vi "Initialize_Msg_Queue_FGV.vi"(8 "error in (no error)":errorcluster, 11 "queue Out":refnum<queue>) -> (0 "error out":errorcluster)   [LabVIEW 2024, in "Barcode_Scanner.lvlib"]
doc: "ThisVI\n---------------------------------\nInitialize_Queue_FGV\n---------------------------------\n-initialize the FGV Message Queue"
uses:
  Barcode_Scanner.lvlib
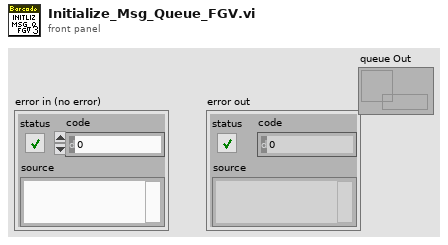
[diagram p1: front panel]
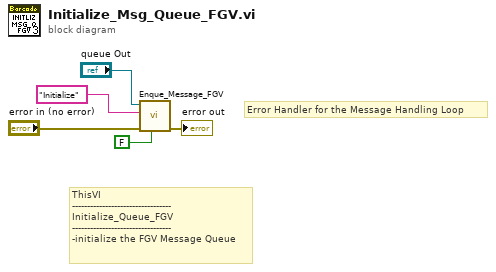
[diagram p0: block diagram]
diagram:
  # "Error Handler for the Message Handling Loop"
  # "ThisVI\n---------------------------------\nInitialize_Queue_FGV\n---------------------------------\n-initialize the FGV Message Queue"
  n1 = call "Enque_Message_FGV.vi"("Priority"=FALSE, "error in (no error)"="error in (no error)", "Message"="Initialize", "queue Out"="queue Out") -> ("error out"=→"error out":errorcluster)  [unwired: 7 in]
